vi "AlGaInPAs_prep_v01.vi"(2 "Debug Mode":bool, 3 "Elapsed Time(s)":dbl, 4 "State":enum16{"Edit", "Start", "Run", "End", "Idle"}(ring), 5 "Argument List In":string[](array[string])) -> (0 "Status Out":string, 1 "Argument List Out":string[](array[string]))   [LabVIEW 2011]
panel:
  out "is OK?":bool
  out "Run started?":bool
  out "prep done?":bool
  out "AsH3?":bool
  out "PH3?":bool
  out "In?":bool
  out "Ga?":bool
  out "Al?":bool
  in  "Prep As":bool caption="Pre-run"
  in  "Prep P":bool caption="Pre-run"
  in  "Prep In":bool caption="Pre-run"
  in  "Prep Ga":bool caption="Pre-run"
  in  "run_time":dbl caption="run time (s)"
  in  "prep_time":dbl caption="pre-run time (s)"
  in  "Prep Al":bool caption="Pre-run"
  in  "Run As":bool caption="Run"
  in  "AsH3 Flow":dbl caption="AsH3 Flow (0-10 sccm)" format="%.2f"
  in  "P Flow":dbl caption="P Flow (0-100 sccm)" format="%.2f"
  in  "Run P":bool caption="Run"
  in  "In Flow":dbl caption="In Flow (0-100 sscm)" format="%.2f"
  in  "Run In":bool caption="Run"
  in  "Run Ga":bool caption="Run"
  in  "Ga Flow":dbl caption="Ga Flow (0-10 sscm)" format="%.2f"
  in  "Run Al":bool caption="Run"
  in  "Al Flow":dbl caption="Al Flow (0-100 sscm)" format="%.2f"
  in  "Cancel":bool
  in  "OK":bool
  out "tTotal(s) 2":dbl
  out "tphase(s)":dbl[](array[numeric])
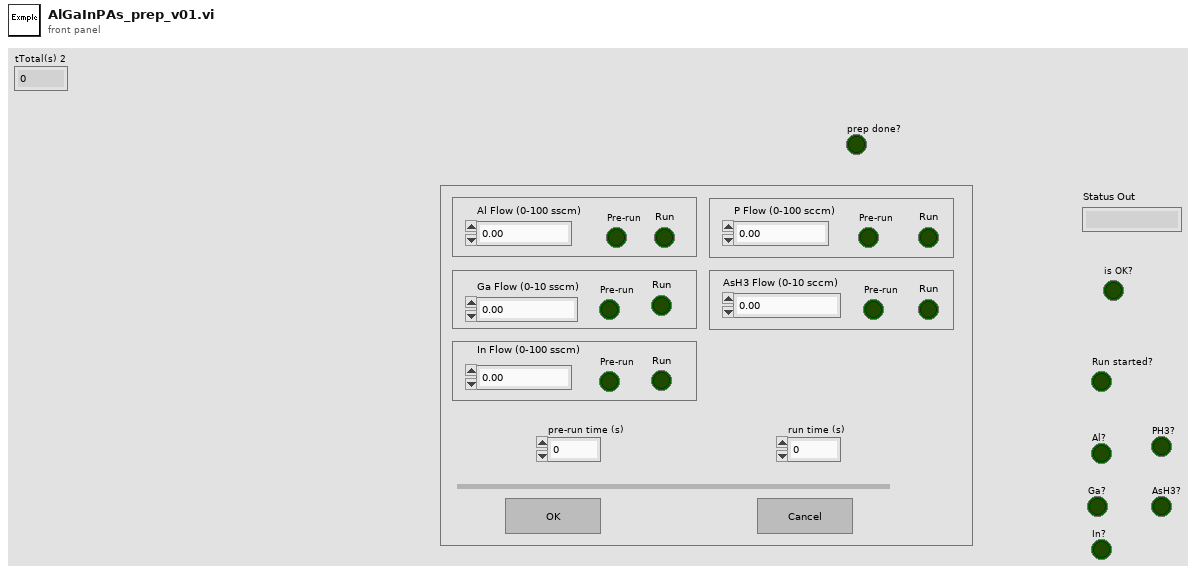
[diagram p1: front panel]
types:
  T1 = enum16{"Discrete", "Continuous", "Instantaneous"}
  T2 = enum32{"Invalid", "Default", "Floating", "Floating/Auto-Hide", "Modal"}
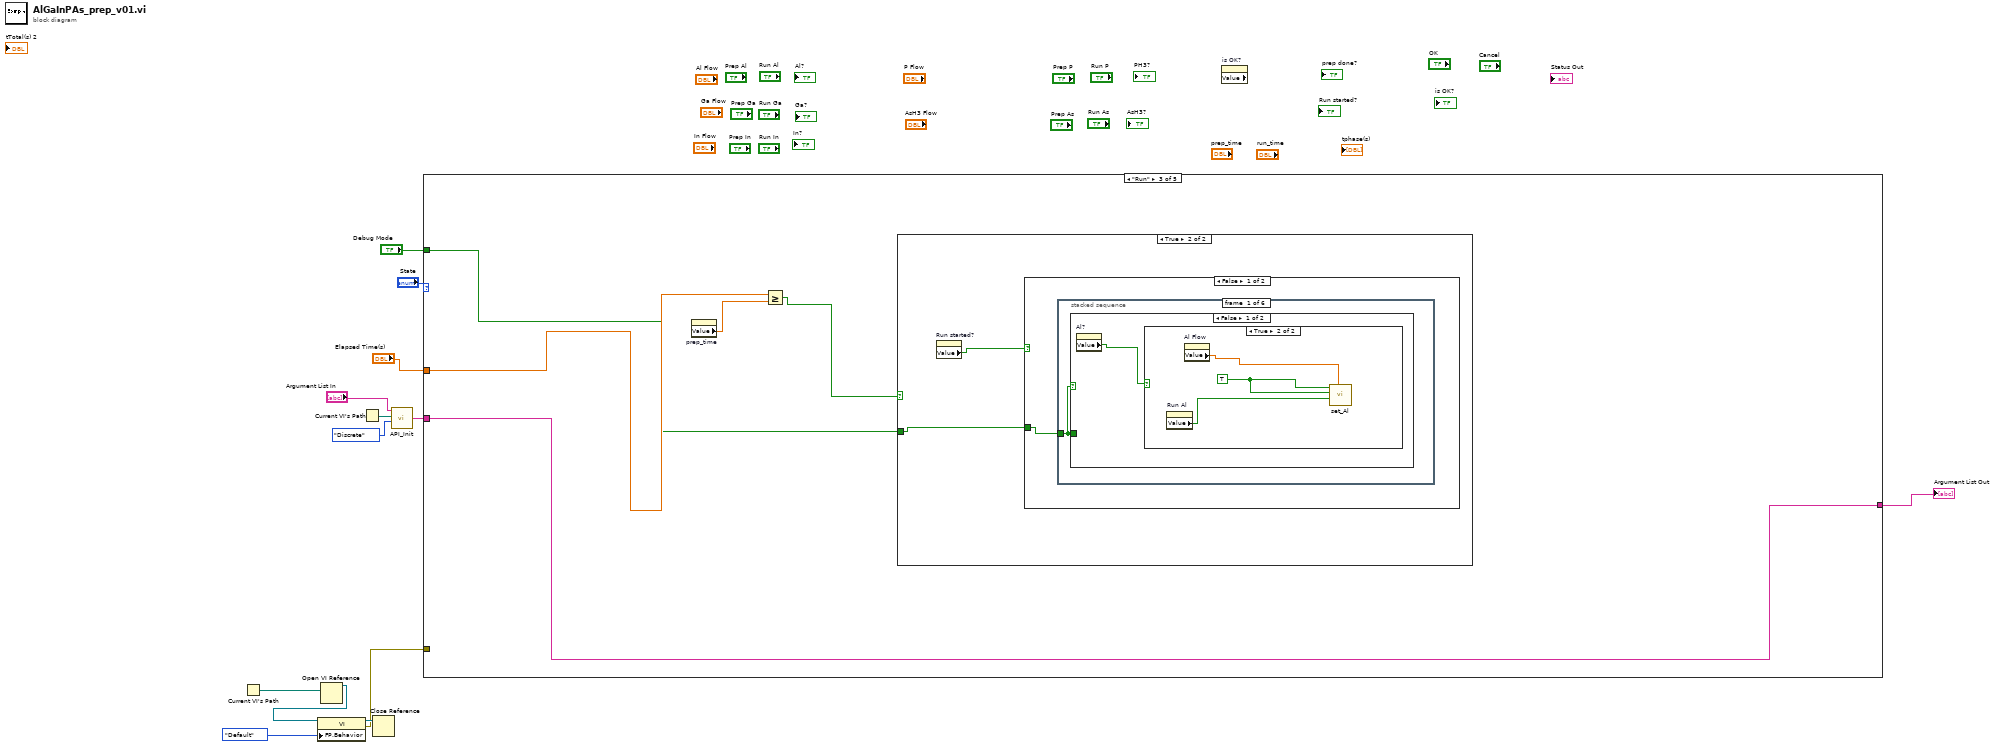
[diagram p0: block diagram]
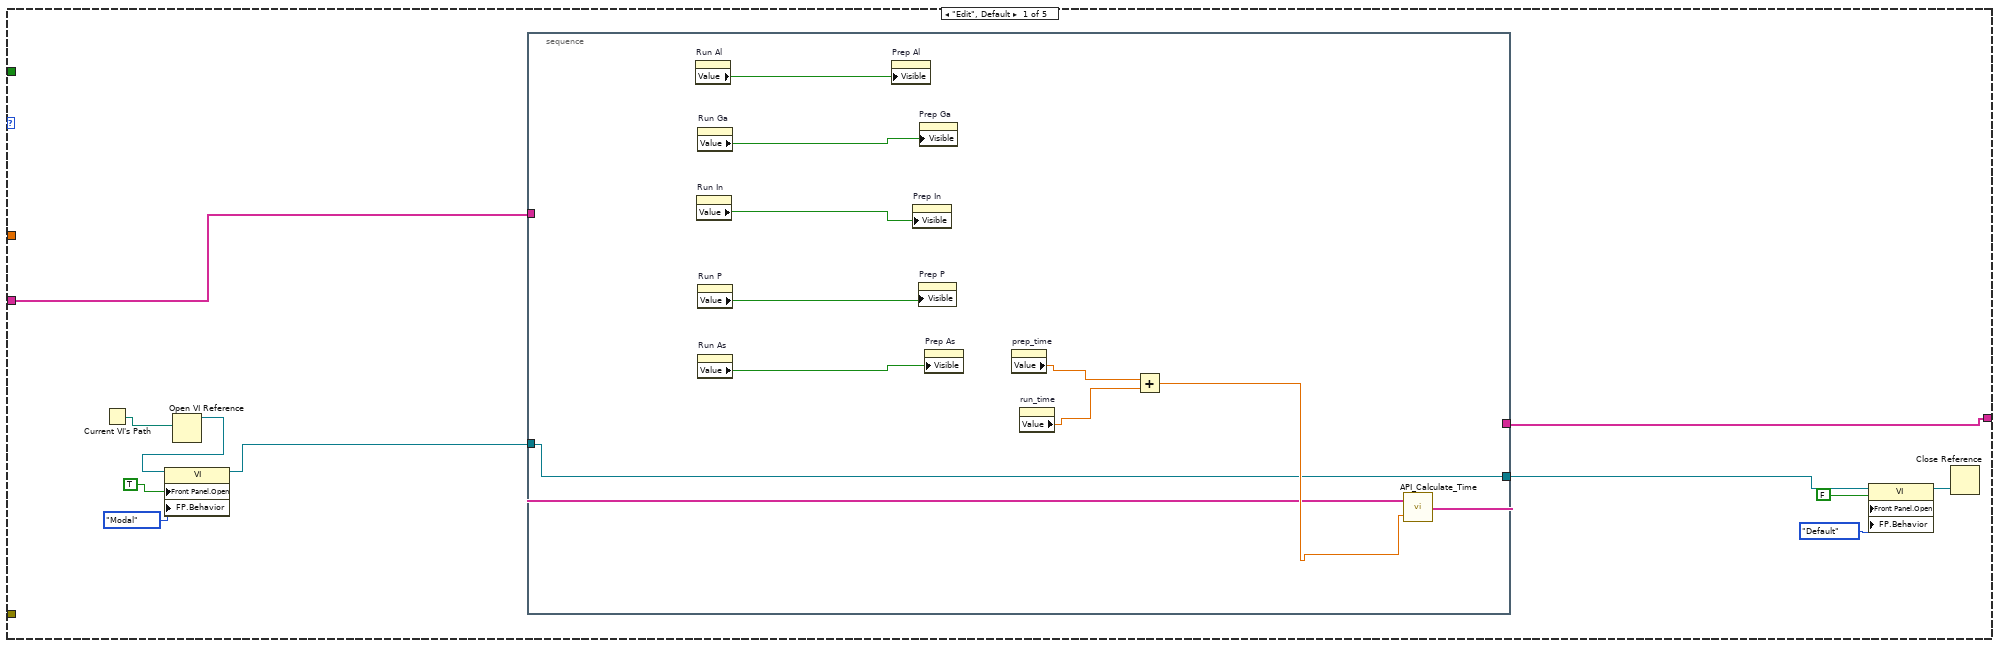
[diagram p2: hidden frame]
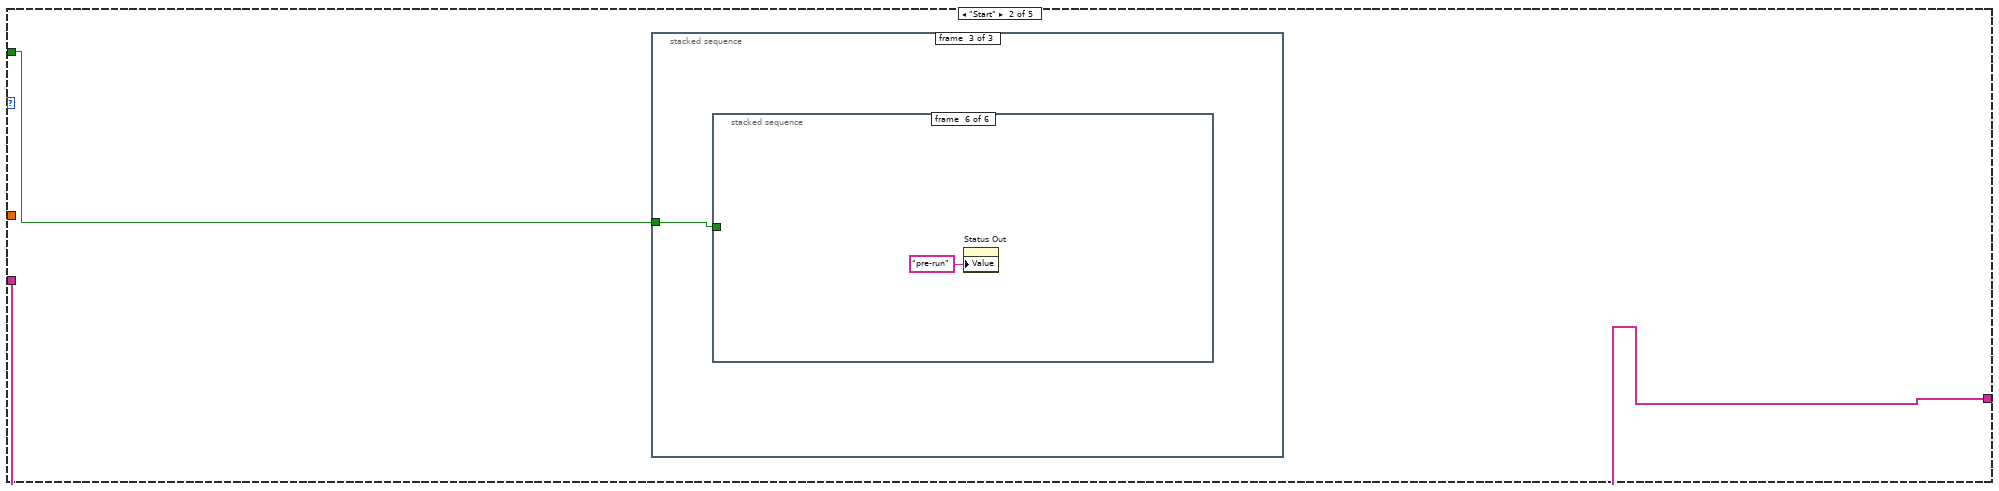
[diagram p3: hidden frame]
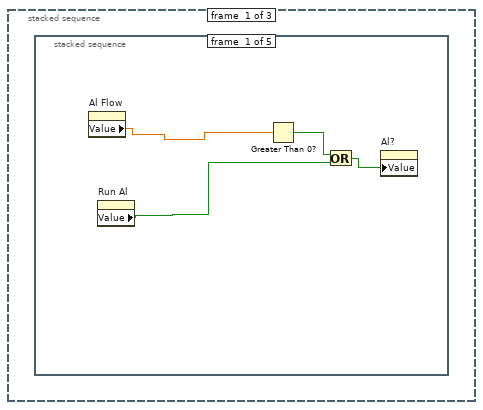
[diagram p4: hidden frame]
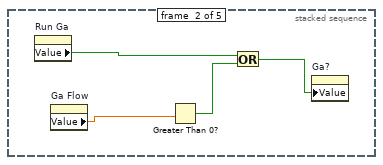
[diagram p5: hidden frame]
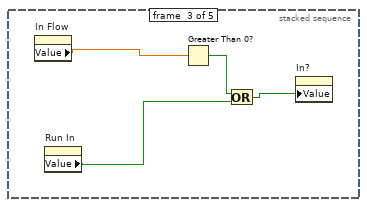
[diagram p6: hidden frame]
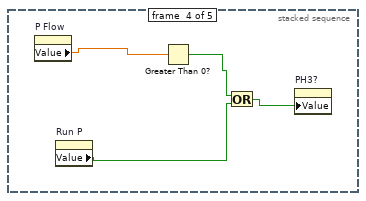
[diagram p7: hidden frame]
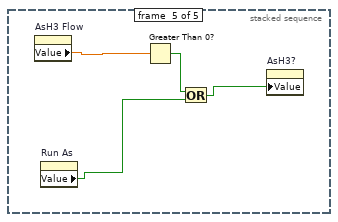
[diagram p8: hidden frame]
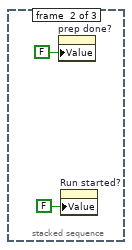
[diagram p9: hidden frame]
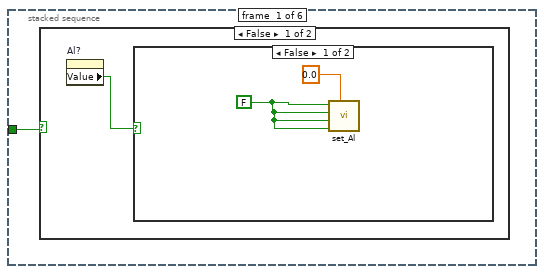
[diagram p10: hidden frame]
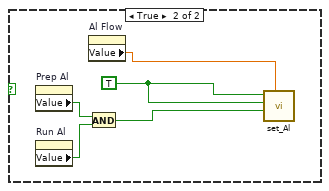
[diagram p11: hidden frame]
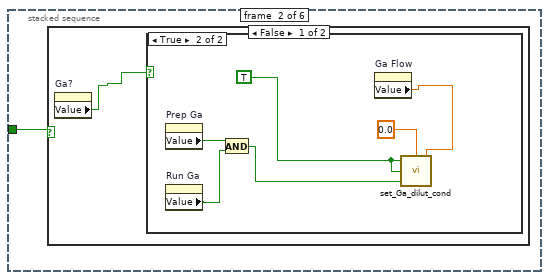
[diagram p13: hidden frame]
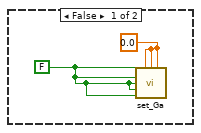
[diagram p14: hidden frame]
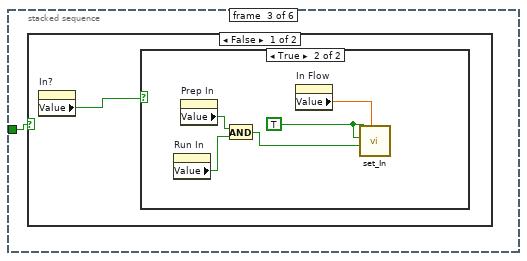
[diagram p16: hidden frame]
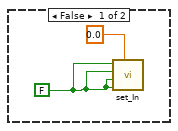
[diagram p17: hidden frame]
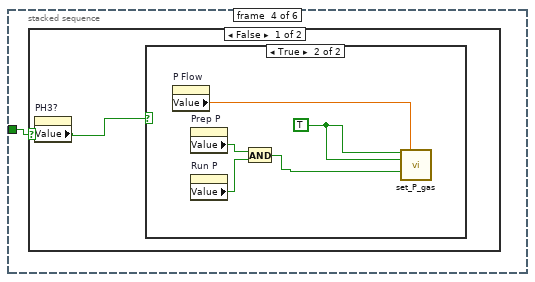
[diagram p19: hidden frame]
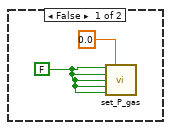
[diagram p20: hidden frame]
diagram:
  n1 = Current VI's Path() -> (path=w9:path)
  n2 = Open VI Reference(vi path=w9) -> (vi reference=w8:refnum<vi>)  [unwired: 1 in, 5 out]
  n3 = property class="VI"(reference=w8, "FP.Behavior"=T2."Default" ("Front Panel Window:Behavior")) -> (reference out=w6:refnum<vi>, error out=w5:errorcluster)  [unwired: 1 in]
  n4 = Current VI's Path() -> (path=w4:path)
  n5 = Close Reference(reference=w6) -> ()  [unwired: 1 in, 1 out]
  n6 = call "API_Init.vi"("API Mode"=T1."Discrete", "VI Path"=w4, "Argument List In"="Argument List In") -> ("Argument List Out"=w1:string[])  [unwired: 1 in]
  n7 = case shown="\"Run\"" "State" {
    tunnel: "Debug Mode" -> [_ w36 w108 _ _]
    tunnel: "Elapsed Time(s)" -> [_ _ w110 _ _]
    tunnel: w1 -> [w14 w37 w112 w154 w155]
    tunnel: [w21 w37 w112 w154 w155] -> w10
    tunnel: w5 -> [_ _ _ _ _]
    frame "Edit", Default {
      n8 = Current VI's Path() -> (path=w19:path)
      n9 = Open VI Reference(vi path=w19) -> (vi reference=w18:refnum<vi>)  [unwired: 1 in, 5 out]
      n10 = property class="VI"(reference=w18, "Front Panel.Open"=TRUE ("Front Panel Window:Open"), "FP.Behavior"=T2."Modal" ("Front Panel Window:Behavior")) -> (reference out=w17:refnum<vi>)  [unwired: 1 in, 1 out]
      n11 = stacked-sequence {
        tunnel: w14 -> [w29]
        tunnel: w17 -> [w25]
        tunnel: [w25] -> w22
        tunnel: [w28] -> w21
        frame #0 {
          n12 = property on="Run Al" class="Bool (strict)"() -> ("Value"=w35:bool)  [unwired: 2 in, 2 out]
          n13 = property on="Run In" class="Bool (strict)"() -> ("Value"=w33:bool)  [unwired: 2 in, 2 out]
          n14 = property on="Run Ga" class="Bool (strict)"() -> ("Value"=w34:bool)  [unwired: 2 in, 2 out]
          n15 = property on="Run P" class="Bool (strict)"() -> ("Value"=w32:bool)  [unwired: 2 in, 2 out]
          n16 = property on="Run As" class="Bool (strict)"() -> ("Value"=w31:bool)  [unwired: 2 in, 2 out]
          n17 = property on="Prep Al" class="Bool (strict)"("Visible"=w35) -> ()  [unwired: 2 in, 2 out]
          n18 = property on="Prep In" class="Bool (strict)"("Visible"=w33) -> ()  [unwired: 2 in, 2 out]
          n19 = property on="Prep P" class="Bool (strict)"("Visible"=w32) -> ()  [unwired: 2 in, 2 out]
          n20 = property on="Prep Ga" class="Bool (strict)"("Visible"=w34) -> ()  [unwired: 2 in, 2 out]
          n21 = property on="Prep As" class="Bool (strict)"("Visible"=w31) -> ()  [unwired: 2 in, 2 out]
          n22 = property on="prep_time" class="DigNum (strict)"() -> ("Value"=w27:dbl)  [unwired: 2 in, 2 out]
          n23 = property on="run_time" class="DigNum (strict)"() -> ("Value"=w26:dbl)  [unwired: 2 in, 2 out]
          n24 = Add(x=w27, y=w26) -> (x+y=w30:dbl)
          n25 = call "API_Calculate_Time.vi"("Time"=w30, "Argument List In"=w29) -> ("Argument List Out"=w28:string[])
        }
      }
      n26 = property class="VI"(reference=w22, "Front Panel.Open"=FALSE ("Front Panel Window:Open"), "FP.Behavior"=T2."Default" ("Front Panel Window:Behavior")) -> (reference out=w23:refnum<vi>)  [unwired: 1 in, 1 out]
      n27 = Close Reference(reference=w23) -> ()  [unwired: 1 in, 1 out]
    }
    frame "Start" {
      n28 = stacked-sequence {
        tunnel: w36 -> [_ _ w60]
        frame #0 {
          n29 = stacked-sequence {
            frame #0 {
              n30 = property on="Al Flow" class="DigNum (strict)"() -> ("Value"=w40:dbl)  [unwired: 2 in, 2 out]
              n31 = property on="Run Al" class="Bool (strict)"() -> ("Value"=w39:bool)  [unwired: 2 in, 2 out]
              n32 = Greater Than 0?(x=w40) -> (x > 0?=w41:bool)
              n33 = Or(x=w41, y=w39) -> (x .or. y?=w38:bool)
              n34 = property on="Al?" class="Bool (strict)"("Value"=w38) -> ()  [unwired: 2 in, 2 out]
            }
            frame #1 {
              n35 = property on="Run Ga" class="Bool (strict)"() -> ("Value"=w43:bool)  [unwired: 2 in, 2 out]
              n36 = property on="Ga Flow" class="DigNum (strict)"() -> ("Value"=w44:dbl)  [unwired: 2 in, 2 out]
              n37 = Greater Than 0?(x=w44) -> (x > 0?=w45:bool)
              n38 = Or(x=w43, y=w45) -> (x .or. y?=w42:bool)
              n39 = property on="Ga?" class="Bool (strict)"("Value"=w42) -> ()  [unwired: 2 in, 2 out]
            }
            frame #2 {
              n40 = property on="In Flow" class="DigNum (strict)"() -> ("Value"=w47:dbl)  [unwired: 2 in, 2 out]
              n41 = property on="Run In" class="Bool (strict)"() -> ("Value"=w48:bool)  [unwired: 2 in, 2 out]
              n42 = Greater Than 0?(x=w47) -> (x > 0?=w49:bool)
              n43 = Or(x=w49, y=w48) -> (x .or. y?=w46:bool)
              n44 = property on="In?" class="Bool (strict)"("Value"=w46) -> ()  [unwired: 2 in, 2 out]
            }
            frame #3 {
              n45 = property on="P Flow" class="DigNum (strict)"() -> ("Value"=w52:dbl)  [unwired: 2 in, 2 out]
              n46 = property on="Run P" class="Bool (strict)"() -> ("Value"=w51:bool)  [unwired: 2 in, 2 out]
              n47 = Greater Than 0?(x=w52) -> (x > 0?=w53:bool)
              n48 = Or(x=w53, y=w51) -> (x .or. y?=w50:bool)
              n49 = property on="PH3?" class="Bool (strict)"("Value"=w50) -> ()  [unwired: 2 in, 2 out]
            }
            frame #4 {
              n50 = property on="AsH3 Flow" class="DigNum (strict)"() -> ("Value"=w56:dbl)  [unwired: 2 in, 2 out]
              n51 = property on="Run As" class="Bool (strict)"() -> ("Value"=w55:bool)  [unwired: 2 in, 2 out]
              n52 = Greater Than 0?(x=w56) -> (x > 0?=w57:bool)
              n53 = Or(x=w57, y=w55) -> (x .or. y?=w54:bool)
              n54 = property on="AsH3?" class="Bool (strict)"("Value"=w54) -> ()  [unwired: 2 in, 2 out]
            }
          }
        }
        frame #1 {
          n55 = property on="prep done?" class="Bool (strict)"("Value"=FALSE ("prep done?")) -> ()  [unwired: 2 in, 2 out]
          n56 = property on="Run started?" class="Bool (strict)"("Value"=FALSE ("Run started?")) -> ()  [unwired: 2 in, 2 out]
        }
        frame #2 {
          n57 = stacked-sequence {
            tunnel: w60 -> [w61 w70 w80 w89 w98 _]
            frame #0 {
              n58 = case shown="False" w61 {
                frame False {
                  n59 = property on="Al?" class="Bool (strict)"() -> ("Value"=w62:bool)  [unwired: 2 in, 2 out]
                  n60 = case shown="False" w62 {
                    frame False {
                      w63 = FALSE ("Al Active")
                      n61 = call "set_Al.vi"("Aluminum Flow"=0.0, "Al Remote"=w63, "Al Run"=w63, "Al Bubbler"=w63, "Al Active"=w63) -> ()  [unwired: 5 out]
                    }
                    frame True {
                      w69 = TRUE ("Al Active")
                      n62 = property on="Prep Al" class="Bool (strict)"() -> ("Value"=w67:bool)  [unwired: 2 in, 2 out]
                      n63 = property on="Run Al" class="Bool (strict)"() -> ("Value"=w66:bool)  [unwired: 2 in, 2 out]
                      n64 = property on="Al Flow" class="DigNum (strict)"() -> ("Value"=w68:dbl)  [unwired: 2 in, 2 out]
                      n65 = And(x=w67, y=w66) -> (x .and. y?=w65:bool)
                      n66 = call "set_Al.vi"("Aluminum Flow"=w68, "Al Run"=w65, "Al Bubbler"=w69, "Al Active"=w69) -> ()  [unwired: 1 in, 5 out]
                    }
                  }
                }
                frame True {
                }
              }
            }
            frame #1 {
              n67 = case shown="False" w70 {
                frame False {
                  n68 = property on="Ga?" class="Bool (strict)"() -> ("Value"=w71:bool)  [unwired: 2 in, 2 out]
                  n69 = case shown="True" w71 {
                    frame False {
                      w73 = FALSE ("Ga Active")
                      w72 = 0.0 ("Ga Flow 1")
                      n70 = call "set_Ga.vi"("Ga Active"=w73, "Ga Flow 3"=w72, "Ga Flow 2"=w72, "Ga Flow 1"=w72, "Ga Bubbler"=w73, "Ga H2 Dilute"=w73, "Ga Run"=w73, "Ga Remote"=w73) -> ()  [unwired: 8 out]
                    }
                    frame True {
                      w79 = TRUE ("Ga Active")
                      n71 = property on="Prep Ga" class="Bool (strict)"() -> ("Value"=w76:bool)  [unwired: 2 in, 2 out]
                      n72 = property on="Run Ga" class="Bool (strict)"() -> ("Value"=w75:bool)  [unwired: 2 in, 2 out]
                      n73 = And(x=w76, y=w75) -> (x .and. y?=w74:bool)
                      n74 = property on="Ga Flow" class="DigNum (strict)"() -> ("Value"=w77:dbl)  [unwired: 2 in, 2 out]
                      n75 = call "set_Ga_dilut_cond.vi"("Ga flow (0-10 sccm)"=w77, "fDilution"=0.0, "Run"=w74, "Bubbler In"=w79, "Active"=w79) -> ()
                    }
                  }
                }
                frame True {
                }
              }
            }
            frame #2 {
              n76 = case shown="False" w80 {
                frame False {
                  n77 = property on="In?" class="Bool (strict)"() -> ("Value"=w81:bool)  [unwired: 2 in, 2 out]
                  n78 = case shown="True" w81 {
                    frame False {
                      w83 = FALSE ("In Remote")
                      n79 = call "set_In.vi"("Indium Flow"=0.0, "In Remote"=w83, "In Run"=w83, "In Bubbler"=w83, "In Active"=w83) -> ()  [unwired: 5 out]
                    }
                    frame True {
                      w88 = TRUE ("In Run")
                      n80 = property on="Run In" class="Bool (strict)"() -> ("Value"=w85:bool)  [unwired: 2 in, 2 out]
                      n81 = property on="Prep In" class="Bool (strict)"() -> ("Value"=w86:bool)  [unwired: 2 in, 2 out]
                      n82 = And(x=w86, y=w85) -> (x .and. y?=w84:bool)
                      n83 = property on="In Flow" class="DigNum (strict)"() -> ("Value"=w87:dbl)  [unwired: 2 in, 2 out]
                      n84 = call "set_In.vi"("Indium Flow"=w87, "In Run"=w84, "In Bubbler"=w88, "In Active"=w88) -> ()  [unwired: 1 in, 5 out]
                    }
                  }
                }
                frame True {
                }
              }
            }
            frame #3 {
              n85 = case shown="False" w89 {
                frame False {
                  n86 = property on="PH3?" class="Bool (strict)"() -> ("Value"=w90:bool)  [unwired: 2 in, 2 out]
                  n87 = case shown="True" w90 {
                    frame False {
                      w91 = FALSE ("P_Gas Active")
                      n88 = call "set_P_gas.vi"("P_Gas Active"=w91, "P_Gas Flow"=0.0, "P_Gas In"=w91, "P_Gas H2 In"=w91, "P_Gas Run"=w91, "P_Gas Remote"=w91) -> ()  [unwired: 10 out]
                    }
                    frame True {
                      w97 = TRUE ("P_Gas Active")
                      n89 = property on="P Flow" class="DigNum (strict)"() -> ("Value"=w96:dbl)  [unwired: 2 in, 2 out]
                      n90 = property on="Prep P" class="Bool (strict)"() -> ("Value"=w95:bool)  [unwired: 2 in, 2 out]
                      n91 = property on="Run P" class="Bool (strict)"() -> ("Value"=w94:bool)  [unwired: 2 in, 2 out]
                      n92 = And(x=w95, y=w94) -> (x .and. y?=w93:bool)
                      n93 = call "set_P_gas.vi"("P_Gas Active"=w97, "P_Gas Flow"=w96, "P_Gas In"=w97, "P_Gas Run"=w93) -> ()  [unwired: 2 in, 10 out]
                    }
                  }
                }
                frame True {
                }
              }
            }
            frame #4 {
              n94 = case shown="False" w98 {
                frame False {
                  n95 = property on="AsH3?" class="Bool (strict)"() -> ("Value"=w99:bool)  [unwired: 2 in, 2 out]
                  n96 = case shown="True" w99 {
                    frame False {
                      w100 = FALSE ("As_Gas Active")
                      n97 = call "set_As_gas.vi"("As_Gas Active"=w100, "As_Gas Flow"=0.0, "As_Gas In"=w100, "As_Gas H2"=w100, "As_Gas Run"=w100, "As_Gas Remote"=w100) -> ()  [unwired: 10 out]
                    }
                    frame True {
                      w106 = TRUE ("As_Gas Active")
                      n98 = property on="Prep As" class="Bool (strict)"() -> ("Value"=w103:bool)  [unwired: 2 in, 2 out]
                      n99 = property on="Run As" class="Bool (strict)"() -> ("Value"=w104:bool)  [unwired: 2 in, 2 out]
                      n100 = property on="AsH3 Flow" class="DigNum (strict)"() -> ("Value"=w105:dbl)  [unwired: 2 in, 2 out]
                      n101 = And(x=w103, y=w104) -> (x .and. y?=w102:bool)
                      n102 = call "set_As_gas.vi"("As_Gas Active"=w106, "As_Gas Flow"=w105, "As_Gas In"=w106, "As_Gas Run"=w102) -> ()  [unwired: 2 in, 10 out]
                    }
                  }
                }
                frame True {
                }
              }
            }
            frame #5 {
              n103 = property on="Status Out" class="Str"("Value"="pre-run" ("Status Out")) -> ()  [unwired: 2 in, 2 out]
            }
          }
        }
      }
    }
    frame "Run" {
      n104 = property on="prep_time" class="DigNum (strict)"() -> ("Value"=w111:dbl)  [unwired: 2 in, 2 out]
      n105 = Greater Or Equal?(x=w110, y=w111) -> (x >= y?=w109:bool)
      n106 = case shown="True" w109 {
        tunnel: w108 -> [_ w113]
        frame False {
        }
        frame True {
          n107 = property on="Run started?" class="Bool (strict)"() -> ("Value"=w114:bool)  [unwired: 2 in, 2 out]
          n108 = case shown="False" w114 {
            tunnel: w113 -> [w115 _]
            frame False {
              n109 = stacked-sequence {
                tunnel: w115 -> [w116 w123 w131 w138 w145 _]
                frame #0 {
                  n110 = case shown="False" w116 {
                    tunnel: w116 -> [_ _]
                    frame False {
                      n111 = property on="Al?" class="Bool (strict)"() -> ("Value"=w117:bool)  [unwired: 2 in, 2 out]
                      n112 = case shown="True" w117 {
                        frame False {
                          w118 = FALSE ("Al Active")
                          n113 = call "set_Al.vi"("Aluminum Flow"=0.0, "Al Remote"=w118, "Al Run"=w118, "Al Bubbler"=w118, "Al Active"=w118) -> ()  [unwired: 5 out]
                        }
                        frame True {
                          w122 = TRUE ("Al Active")
                          n114 = property on="Run Al" class="Bool (strict)"() -> ("Value"=w120:bool)  [unwired: 2 in, 2 out]
                          n115 = property on="Al Flow" class="DigNum (strict)"() -> ("Value"=w121:dbl)  [unwired: 2 in, 2 out]
                          n116 = call "set_Al.vi"("Aluminum Flow"=w121, "Al Run"=w120, "Al Bubbler"=w122, "Al Active"=w122) -> ()  [unwired: 1 in, 5 out]
                        }
                      }
                    }
                    frame True {
                    }
                  }
                }
                frame #1 {
                  n117 = case shown="False" w123 {
                    frame False {
                      n118 = property on="Ga?" class="Bool (strict)"() -> ("Value"=w124:bool)  [unwired: 2 in, 2 out]
                      n119 = case shown="True" w124 {
                        frame False {
                          w126 = FALSE ("Ga Active")
                          w125 = 0.0 ("Ga Flow 1")
                          n120 = call "set_Ga.vi"("Ga Active"=w126, "Ga Flow 3"=w125, "Ga Flow 2"=w125, "Ga Flow 1"=w125, "Ga Bubbler"=w126, "Ga H2 Dilute"=w126, "Ga Run"=w126, "Ga Remote"=w126) -> ()  [unwired: 8 out]
                        }
                        frame True {
                          w130 = TRUE ("Ga Active")
                          n121 = property on="Run Ga" class="Bool (strict)"() -> ("Value"=w128:bool)  [unwired: 2 in, 2 out]
                          n122 = property on="Ga Flow" class="DigNum (strict)"() -> ("Value"=w127:dbl)  [unwired: 2 in, 2 out]
                          n123 = call "set_Ga_dilut_cond.vi"("Ga flow (0-10 sccm)"=w127, "fDilution"=0.0, "Run"=w128, "Bubbler In"=w130, "Active"=w130) -> ()
                        }
                      }
                    }
                    frame True {
                    }
                  }
                }
                frame #2 {
                  n124 = case shown="False" w131 {
                    frame False {
                      n125 = property on="In?" class="Bool (strict)"() -> ("Value"=w132:bool)  [unwired: 2 in, 2 out]
                      n126 = case shown="True" w132 {
                        frame False {
                          w134 = FALSE ("In Remote")
                          n127 = call "set_In.vi"("Indium Flow"=0.0, "In Remote"=w134, "In Run"=w134, "In Bubbler"=w134, "In Active"=w134) -> ()  [unwired: 5 out]
                        }
                        frame True {
                          w137 = TRUE ("In Run")
                          n128 = property on="Run In" class="Bool (strict)"() -> ("Value"=w135:bool)  [unwired: 2 in, 2 out]
                          n129 = property on="In Flow" class="DigNum (strict)"() -> ("Value"=w136:dbl)  [unwired: 2 in, 2 out]
                          n130 = call "set_In.vi"("Indium Flow"=w136, "In Run"=w135, "In Bubbler"=w137, "In Active"=w137) -> ()  [unwired: 1 in, 5 out]
                        }
                      }
                    }
                    frame True {
                    }
                  }
                }
                frame #3 {
                  n131 = case shown="False" w138 {
                    frame False {
                      n132 = property on="PH3?" class="Bool (strict)"() -> ("Value"=w139:bool)  [unwired: 2 in, 2 out]
                      n133 = case shown="False" w139 {
                        frame False {
                          w140 = FALSE ("P_Gas Active")
                          n134 = call "set_P_gas.vi"("P_Gas Active"=w140, "P_Gas Flow"=0.0, "P_Gas In"=w140, "P_Gas H2 In"=w140, "P_Gas Run"=w140, "P_Gas Remote"=w140) -> ()  [unwired: 10 out]
                        }
                        frame True {
                          w144 = TRUE ("P_Gas Active")
                          n135 = property on="Run P" class="Bool (strict)"() -> ("Value"=w142:bool)  [unwired: 2 in, 2 out]
                          n136 = property on="P Flow" class="DigNum (strict)"() -> ("Value"=w143:dbl)  [unwired: 2 in, 2 out]
                          n137 = call "set_P_gas.vi"("P_Gas Active"=w144, "P_Gas Flow"=w143, "P_Gas In"=w144, "P_Gas Run"=w142) -> ()  [unwired: 2 in, 10 out]
                        }
                      }
                    }
                    frame True {
                    }
                  }
                }
                frame #4 {
                  n138 = case shown="False" w145 {
                    frame False {
                      n139 = property on="AsH3?" class="Bool (strict)"() -> ("Value"=w146:bool)  [unwired: 2 in, 2 out]
                      n140 = case shown="True" w146 {
                        frame False {
                          w147 = FALSE ("As_Gas Active")
                          n141 = call "set_As_gas.vi"("As_Gas Active"=w147, "As_Gas Flow"=0.0, "As_Gas In"=w147, "As_Gas H2"=w147, "As_Gas Run"=w147, "As_Gas Remote"=w147) -> ()  [unwired: 10 out]
                        }
                        frame True {
                          w150 = TRUE ("As_Gas Active")
                          n142 = property on="AsH3 Flow" class="DigNum (strict)"() -> ("Value"=w151:dbl)  [unwired: 2 in, 2 out]
                          n143 = property on="Run As" class="Bool (strict)"() -> ("Value"=w149:bool)  [unwired: 2 in, 2 out]
                          n144 = call "set_As_gas.vi"("As_Gas Active"=w150, "As_Gas Flow"=w151, "As_Gas In"=w150, "As_Gas Run"=w149) -> ()  [unwired: 2 in, 10 out]
                        }
                      }
                    }
                    frame True {
                    }
                  }
                }
                frame #5 {
                  n145 = property on="Run started?" class="Bool (strict)"("Value"=TRUE ("Run started?")) -> ()  [unwired: 2 in, 2 out]
                  n146 = property on="Status Out" class="Str"("Value"="run started" ("Status Out")) -> ()  [unwired: 2 in, 2 out]
                }
              }
            }
            frame True {
            }
          }
        }
      }
    }
    frame "End" {
    }
    frame "Idle" {
    }
  }
  "Argument List Out" <- w10
  n147 = property on="is OK?" class="Bool (strict)" props=["Value"]() -> ()  [unwired: 2 in, 3 out]
